vi "VI Tree.vi"   [LabVIEW 2010, in "California Instruments iX Series.lvlib"]
doc: "This is the instrument driver for the California Instruments iX Series. The VI Tree displays all the user-callable VIs of the instrument driver in an organized table."
uses:
  <instrlib>/California Instruments iX Series/California Instruments iX Series.lvlib
  <instrlib>/California Instruments iX Series/Public/Data/Read Single Current Measurement.vi
  <instrlib>/California Instruments iX Series/Public/Data/Read Single Voltage Measurement.vi
panel:
  # "(c) 2009 National Instruments.  ALL RIGHTS RESERVED."
  # "SEE DIAGRAM\nFOR VI TREE."
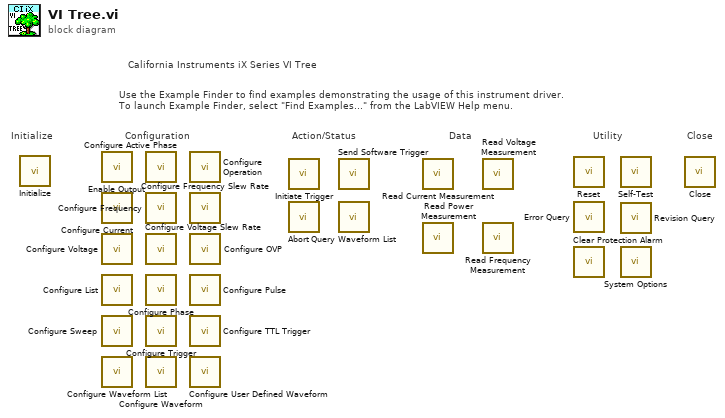
[diagram p0: block diagram]
diagram:
  # "California Instruments iX Series VI Tree"
  # "Use the Example Finder to find examples demonstrating the usage of this instrument driver.\nTo launch Example Finder, select \"Find Examples...\" from the LabVIEW Help menu."
  # "Configuration"
  # "Utility"
  # "Data"
  # "Action/Status"
  # "Close"
  # "Initialize"
  n1 = call <instrlib>:"Initialize.vi"() -> ()  [unwired: 10 in, 2 out]
  n2 = call <instrlib>:"Enable Output.vi"() -> ()  [unwired: 10 in, 2 out]
  n3 = call <instrlib>:"Configure Current.vi"() -> ()  [unwired: 14 in, 2 out]
  n4 = call <instrlib>:"Configure Voltage.vi"() -> ()  [unwired: 14 in, 2 out]
  n5 = call <instrlib>:"Configure List.vi"() -> ()  [unwired: 10 in, 2 out]
  n6 = call <instrlib>:"Configure Sweep.vi"() -> ()  [unwired: 10 in, 2 out]
  n7 = call <instrlib>:"Configure Waveform List.vi"() -> ()  [unwired: 10 in, 2 out]
  n8 = call <instrlib>:"Configure Active Phase.vi"() -> ()  [unwired: 14 in, 2 out]
  n9 = call <instrlib>:"Configure Frequency.vi"() -> ()  [unwired: 14 in, 2 out]
  n10 = call <instrlib>:"Configure Voltage Slew Rate.vi"() -> ()  [unwired: 14 in, 2 out]
  n11 = call <instrlib>:"Configure Phase.vi"() -> ()  [unwired: 14 in, 2 out]
  n12 = call <instrlib>:"Configure Trigger.vi"() -> ()  [unwired: 14 in, 2 out]
  n13 = call <instrlib>:"Configure Waveform.vi"() -> ()  [unwired: 14 in, 2 out]
  n14 = call <instrlib>:"Configure Operation.vi"() -> ()  [unwired: 10 in, 2 out]
  n15 = call <instrlib>:"Configure Frequency Slew Rate.vi"() -> ()  [unwired: 14 in, 2 out]
  n16 = call <instrlib>:"Configure OVP.vi"() -> ()  [unwired: 10 in, 2 out]
  n17 = call <instrlib>:"Configure Pulse.vi"() -> ()  [unwired: 14 in, 2 out]
  n18 = call <instrlib>:"Configure TTL Trigger.vi"() -> ()  [unwired: 14 in, 2 out]
  n19 = call <instrlib>:"Configure User Defined Waveform.vi"() -> ()  [unwired: 14 in, 2 out]
  n20 = call <instrlib>:"Initiate Trigger.vi"() -> ()  [unwired: 10 in, 2 out]
  n21 = call <instrlib>:"Abort.vi"() -> ()  [unwired: 10 in, 2 out]
  n22 = call <instrlib>:"Send Software Trigger.vi"() -> ()  [unwired: 10 in, 2 out]
  n23 = call <instrlib>:"Query Waveform List.vi"() -> ()  [unwired: 9 in, 3 out]
  n24 = call-poly <instrlib>:"Read Current Measurement.vi"() -> ()  [unwired: 9 in, 3 out]
  n25 = call <instrlib>:"Read Power Measurement.vi"() -> ()  [unwired: 9 in, 3 out]
  n26 = call-poly <instrlib>:"Read Voltage Measurement.vi"() -> ()  [unwired: 9 in, 3 out]
  n27 = call <instrlib>:"Read Frequency Measurement.vi"() -> ()  [unwired: 9 in, 3 out]
  n28 = call <instrlib>:"Reset.vi"() -> ()  [unwired: 10 in, 2 out]
  n29 = call <instrlib>:"Error Query.vi"() -> ()  [unwired: 8 in, 4 out]
  n30 = call <instrlib>:"Clear Protection Alarm.vi"() -> ()  [unwired: 10 in, 2 out]
  n31 = call <instrlib>:"Self-Test.vi"() -> ()  [unwired: 8 in, 4 out]
  n32 = call <instrlib>:"Revision Query.vi"() -> ()  [unwired: 8 in, 4 out]
  n33 = call <instrlib>:"System Options.vi"() -> ()  [unwired: 14 in, 2 out]
  n34 = call <instrlib>:"Close.vi"() -> ()  [unwired: 11 in, 1 out]
